vi "dsdll_capture_wave_byte_array.vi"(8 "error in":errorcluster, 10 "samples count in":u32, 11 "dsdll instance in":T2={"dsdll path"=path "E:/LVprog/DirectSoundDLL/dsdll.dll", "dsdll handle"=[], "output devices"=[], "capture devices"=[]}) -> (0 "error out":errorcluster, 1 "wave data":u8[](array[numeric]), 2 "samples count out":u32, 3 "dsdll instance out":T2, 4 "channels count":u16, 5 "time stamp [s]":dbl, 6 "format":T1, 7 "byte count out":u32)   [LabVIEW 2018, in "dsdll.lvlib"]
doc: "Call this to capture waveform of specified length.\n\nThis VI si synchronous so it won't return untill entire waveform is recorded."
uses:
  dsdll.lvlib
  dsdll_instance.ctl
  dsdll_device_record.ctl
  dsdll_sample_format.ctl
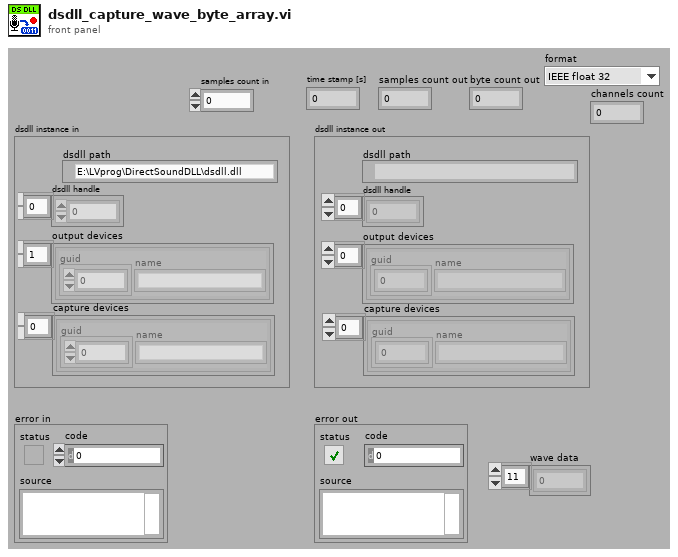
[diagram p1: front panel]
types:
  T1 = typedef "dsdll.lvlib/dsdll_sample_format.ctl" = enum16{"IEEE float 32", "PCM 16 bit"}
  T2 = typedef "dsdll.lvlib/dsdll_instance.ctl" = cluster{"dsdll path":path, "dsdll handle":u8[], "output devices":T3[], "capture devices":T3[]}
  T3 = typedef "dsdll.lvlib/dsdll_device_record.ctl" = cluster{"guid":u8[], "name":string}
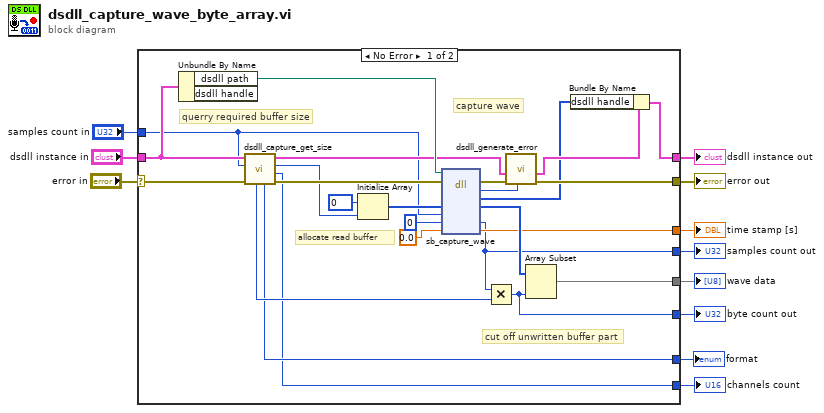
[diagram p0: block diagram]
diagram:
  n1 = case shown="No Error" "error in" {
    selector: "error in" -> [w20 w37]
    tunnel: "dsdll instance in" -> [w17 w38]
    tunnel: [w34 w37] -> w10
    tunnel: [w31 w38] -> w11
    tunnel: "samples count in" -> [w16 _]
    tunnel: [w25 _] -> w6
    tunnel: [w21 _] -> w5
    tunnel: [w24 _] -> w4
    tunnel: [w23 _] -> w3
    tunnel: [w13 _] -> w2
    tunnel: [w12 _] -> w1
    frame No Error {
      # "cut off unwritten buffer part"
      # "allocate read buffer"
      # "querry required buffer size"
      # "capture wave"
      n2 = Unbundle By Name(w17) -> ("dsdll path"=w22:path)  [unwired: 1 out]
      n3 = call "dsdll_capture_get_size.vi"("error in"=w20, "samples count"=w16, "dsdll instance in"=w17) -> ("error out"=w19:errorcluster, "channels count"=w12:u16, "capture buffer size [B]"=w15:u32, "dsdll instance out"=w18:T2, "format"=w13:T1, "total sample size [B]"=w14:i32)  [unwired: 3 in]
      n4 = Initialize Array(u8 0 ("bsize"), w15) -> (w29:u8[])
      n5 = dll-call lib="dsdll.dll" fn="sb_capture_wave" ("sb_get_handle_size()")(path in=w22, error in=w19, "data"=w29, "count"=w16, "read"=u32 0, "time_stamp"=0.0) -> (error out=w36:errorcluster, "error"=w35:i32, "handle"=w32:u8[], "data"=w26:u8[], "read"=w21:u32, "time_stamp"=w25:dbl)  [unwired: 3 in, 1 out]
      n6 = Multiply(x=w21, y=w14) -> (x*y=w24:u32)
      n7 = call "dsdll_generate_error.vi"("error code"=w35, "error in"=w36, "dsdll instance in"=w18) -> ("error out"=w34:errorcluster, "dsdll instance out"=w33:T2)  [unwired: 6 in, 1 out]
      n8 = Array Subset(array=w26, length=w24) -> (w23:u8[])  [unwired: 1 in]
      n9 = Bundle By Name(cluster=w33, "dsdll handle"=w32) -> (w31:T2)
    }
    frame Error {
    }
  }
  "error out" <- w10
  "dsdll instance out" <- w11
  "wave data" <- w3
  "time stamp [s]" <- w6
  "samples count out" <- w5
  "byte count out" <- w4
  "format" <- w2
  "channels count" <- w1
